vi "Load.vi"(8 "error in (no error)":errorcluster, 11 "Gantry In":refnum<class "Gantry Class.lvclass">) -> (0 "error out":errorcluster, 3 "CameraTool out":refnum<class "CameraTool Class.lvclass">)   [LabVIEW 2011, in "CameraTool Class.lvclass"]
uses:
  CameraTool Class.lvclass
  Gantry Class/Gantry Class.lvclass
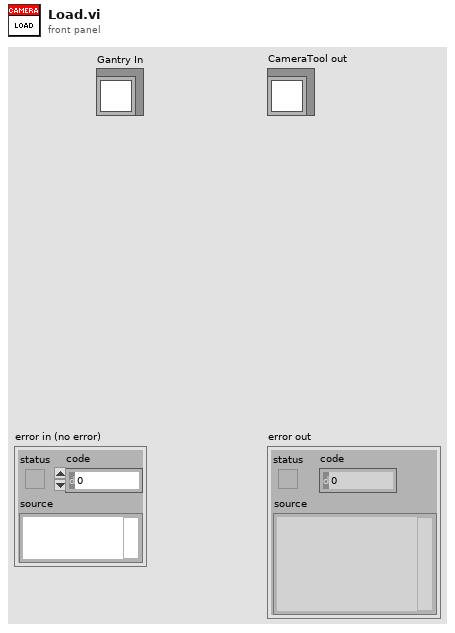
[diagram p1: front panel]
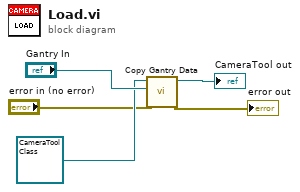
[diagram p0: block diagram]
diagram:
  n1 = call "Copy Gantry Data.vi"("error in (no error)"="error in (no error)", "Gantry Source"="Gantry In", "Gantry Dest"=refnum<class "CameraTool Class.lvclass"> refnum ("CameraTool Class in")) -> ("error out"=→"error out":errorcluster, "Gantry Result"=→"CameraTool out":refnum<class "CameraTool Class.lvclass">)  [unwired: 7 in]
